vi "LEDflash.vi"   [LabVIEW 2014]
uses:
  <vilib>/DAQmx/write.llb/DAQmx Write (Digital Bool 1Line 1Point).vi
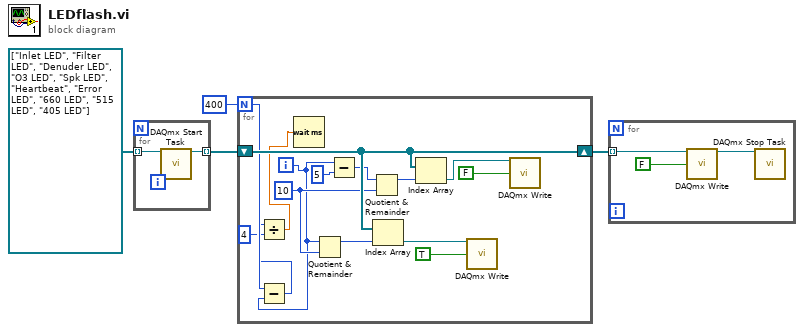
[diagram p0: block diagram]
diagram:
  n1 = for {
    tunnel: refnum<k21>[] ["Inlet LED", "Filter LED", "Denuder LED", "O3 LED", "Spk LED", "Heartbeat", "Error LED", "660 LED", "515 LED", "405 LED"] -> [w6] mode=indexing
    tunnel: [w5] -> w3 mode=indexing
    n2 = call <vilib>:"DAQmx Start Task.vi"("task/channels in"=w6) -> ("task out"=w5:refnum<k21>)  [unwired: 13 in, 1 out]
  }
  n3 = for {
    N: 400 -> [w11]
    shift-right: [w17] -> w2
    shift-left: w3 -> [w17]
    i -> [w10]
    w15 = 10 ("y")
    n4 = Subtract(x=w11, y=w10) -> (x-y=w9:i32)
    n5 = Divide(x=w9, y=4) -> (x/y=w7:dbl)
    n6 = Wait (ms)(milliseconds to wait=w7) -> ()  [unwired: 1 out]
    n7 = Quotient & Remainder(x=w10, y=w15) -> (x-y*floor(x/y)=w19:i32)  [unwired: 1 out]
    n8 = Subtract(x=w10, y=5) -> (x-y=w16:i32)
    n9 = Quotient & Remainder(x=w16, y=w15) -> (x-y*floor(x/y)=w14:i32)  [unwired: 1 out]
    n10 = Index Array(array=w17, index=w19) -> (element=w18:refnum<k21>)
    n11 = Index Array(array=w17, index=w14) -> (element=w13:refnum<k21>)
    n12 = call-poly <vilib>:"DAQmx Write.vi"("task/channels in"=w18, "data"=TRUE) -> ()  [unwired: 11 in, 3 out]
    n13 = call-poly <vilib>:"DAQmx Write.vi"("task/channels in"=w13, "data"=FALSE) -> ()  [unwired: 11 in, 3 out]
  }
  n14 = for {
    tunnel: w2 -> [w23] mode=indexing
    n15 = call-poly <vilib>:"DAQmx Write.vi"("task/channels in"=w23, "data"=FALSE) -> ("task out"=w22:refnum<k21>)  [unwired: 11 in, 2 out]
    n16 = call <vilib>:"DAQmx Stop Task.vi"("task/channels in"=w22) -> ()  [unwired: 13 in, 2 out]
  }
